vi "everything.vi"   [LabVIEW 2011]
uses:
  gfitsio.lvlib
  cfitsio-hdutypes.ctl
  gfitsio-error-codes.ctl
  gfitsio-refnum.ctl
  cfitsio-bitpix.ctl
types:
  T1 = typedef "gfitsio.lvlib/gfitsio-refnum.ctl" = refnum<k1>
  T2 = typedef "gfitsio.lvlib/cfitsio-hdutypes.ctl" = i32
  T3 = typedef "gfitsio.lvlib/gfitsio-error-codes.ctl" = i32
  T4 = typedef "gfitsio.lvlib/cfitsio-bitpix.ctl" = i32
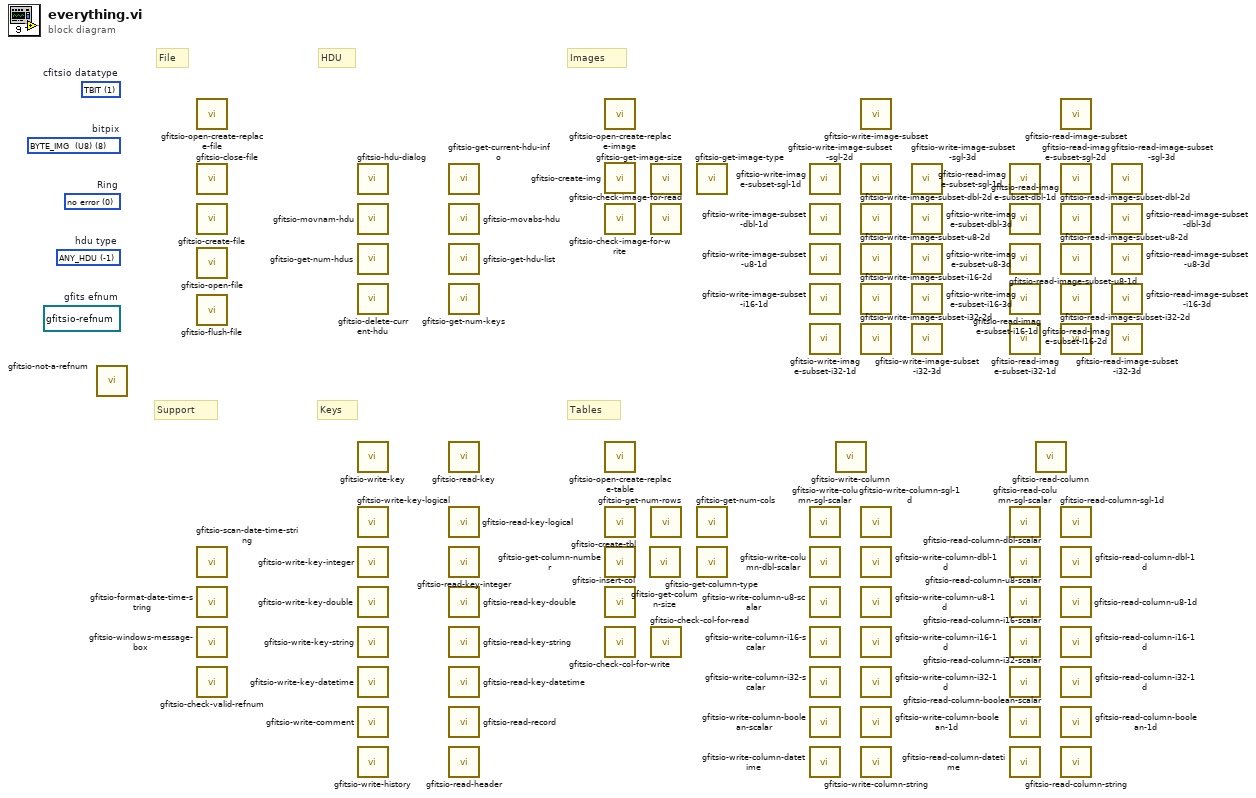
[diagram p0: block diagram]
diagram:
  (unwired) T1 refnum items=["GFITSIO"]  # gfits efnum
  (unwired) T2 -1 items=["ANY_HDU"=-1, "IMAGE_HDU"=0, "ASCII_TBL"=1, "BINARY_TBL"=2]  # hdu type
  (unwired) T3 0 items=["no error"=0, "dimensionality conflict"=5001, "fpixel out of image bounds"=5002, "lpixel out of image bounds"=5003, "increment size larger than image"=5004, "increment must be greater than zero"=5005, "fpixel must specify lower left corner"=5006, "named HDU not found"=5007, "specified row is past the end of the table"=5008, "wrong number of elements for column"=5009, "column is not scalar"=5010, "duplicate HDU name"=5011, "invalid table type"=5012]  # Ring
  (unwired) T4 8 items=["<invalid type>"=0, "BYTE_IMG  (U8)"=8, "SHORT_IMG  (I16)"=16, "USHORT_IMG  (U16)"=20, "LONG_IMG  (I32)"=32, "ULONG_IMG  (U32)"=40, "FLOAT_IMG  (SGL)"=-32, "DOUBLE_IMG  (DBL)"=-64]  # bitpix
  (unwired) T2 1 items=["TBIT"=1, "TBYTE  (U8)"=11, "TSBYTE  (I8)"=12, "TLOGICAL"=14, "TSTRING"=16, "TUSHORT  (U16)"=20, "TSHORT  (I16)"=21, "TUINT"=31, "TULONG  (U32)"=40, "TLONG  (I32)"=41, "TFLOAT  (SGL)"=42, "TLONGLONG  (I64)"=81, "TDOUBLE  (DBL)"=82, "TCOMPLEX  (CSG)"=83, "TDOUBLECOMPLEX  (CDB)"=163]  # cfitsio datatype
  # "Tables"
  # "Keys"
  # "Support"
  # "Images"
  # "HDU"
  # "File"
  n1 = call "gfitsio-not-a-refnum.vi"() -> ()  [unwired: 1 out]
  n2 = call "gfitsio-open-create-replace-file.vi"() -> ()  [unwired: 9 in, 3 out]
  n3 = call "gfitsio-close-file.vi"() -> ()  [unwired: 10 in, 2 out]
  n4 = call "gfitsio-create-file.vi"() -> ()  [unwired: 10 in, 2 out]
  n5 = call "gfitsio-open-file.vi"() -> ()  [unwired: 10 in, 2 out]
  n6 = call "gfitsio-flush-file.vi"() -> ()  [unwired: 10 in, 2 out]
  n7 = call "gfitsio-scan-date-time-string.vi"() -> ()  [unwired: 10 in, 2 out]
  n8 = call "gfitsio-format-date-time-string.vi"() -> ()  [unwired: 11 in, 1 out]
  n9 = call "gfitsio-windows-message-box.vi"() -> ()  [unwired: 11 in, 1 out]
  n10 = call "gfitsio-check-valid-refnum.vi"() -> ()  [unwired: 5 in, 1 out]
  n11 = call "gfitsio-hdu-dialog.vi"() -> ()  [unwired: 6 in, 6 out]
  n12 = call "gfitsio-movnam-hdu.vi"() -> ()  [unwired: 10 in, 2 out]
  n13 = call "gfitsio-get-num-hdus.vi"() -> ()  [unwired: 9 in, 3 out]
  n14 = call "gfitsio-delete-current-hdu.vi"() -> ()  [unwired: 10 in, 2 out]
  n15 = call-poly "gfitsio-write-key.vi"() -> ()  [unwired: 10 in, 2 out]
  n16 = call "gfitsio-write-key-logical.vi"() -> ()  [unwired: 10 in, 2 out]
  n17 = call "gfitsio-write-key-integer.vi"() -> ()  [unwired: 10 in, 2 out]
  n18 = call "gfitsio-write-key-double.vi"() -> ()  [unwired: 10 in, 2 out]
  n19 = call "gfitsio-write-key-string.vi"() -> ()  [unwired: 10 in, 2 out]
  n20 = call "gfitsio-write-key-datetime.vi"() -> ()  [unwired: 10 in, 2 out]
  n21 = call "gfitsio-write-comment.vi"() -> ()  [unwired: 10 in, 2 out]
  n22 = call "gfitsio-write-history.vi"() -> ()  [unwired: 10 in, 2 out]
  n23 = call "gfitsio-get-current-hdu-info.vi"() -> ()  [unwired: 7 in, 5 out]
  n24 = call "gfitsio-movabs-hdu.vi"() -> ()  [unwired: 9 in, 3 out]
  n25 = call "gfitsio-get-hdu-list.vi"() -> ()  [unwired: 8 in, 4 out]
  n26 = call "gfitsio-get-num-keys.vi"() -> ()  [unwired: 9 in, 3 out]
  n27 = call-poly "gfitsio-read-key.vi"() -> ()  [unwired: 7 in, 5 out]
  n28 = call "gfitsio-read-key-logical.vi"() -> ()  [unwired: 8 in, 4 out]
  n29 = call "gfitsio-read-key-integer.vi"() -> ()  [unwired: 7 in, 5 out]
  n30 = call "gfitsio-read-key-double.vi"() -> ()  [unwired: 7 in, 5 out]
  n31 = call "gfitsio-read-key-string.vi"() -> ()  [unwired: 8 in, 4 out]
  n32 = call "gfitsio-read-key-datetime.vi"() -> ()  [unwired: 8 in, 4 out]
  n33 = call "gfitsio-read-record.vi"() -> ()  [unwired: 9 in, 3 out]
  n34 = call "gfitsio-read-header.vi"() -> ()  [unwired: 9 in, 3 out]
  n35 = call "gfitsio-open-create-replace-image.vi"() -> ()  [unwired: 9 in, 3 out]
  n36 = call "gfitsio-create-img.vi"() -> ()  [unwired: 10 in, 2 out]
  n37 = call "gfitsio-check-image-for-write.vi"() -> ()  [unwired: 10 in, 2 out]
  n38 = call "gfitsio-open-create-replace-table.vi"() -> ()  [unwired: 9 in, 3 out]
  n39 = call "gfitsio-create-tbl.vi"() -> ()  [unwired: 10 in, 2 out]
  n40 = call "gfitsio-get-column-number.vi"() -> ()  [unwired: 9 in, 3 out]
  n41 = call "gfitsio-insert-col.vi"() -> ()  [unwired: 10 in, 2 out]
  n42 = call "gfitsio-check-col-for-write.vi"() -> ()  [unwired: 9 in, 3 out]
  n43 = call "gfitsio-get-column-size.vi"() -> ()  [unwired: 8 in, 4 out]
  n44 = call "gfitsio-get-image-size.vi"() -> ()  [unwired: 8 in, 4 out]
  n45 = call "gfitsio-check-image-for-read.vi"() -> ()  [unwired: 9 in, 3 out]
  n46 = call "gfitsio-get-num-rows.vi"() -> ()  [unwired: 9 in, 3 out]
  n47 = call "gfitsio-check-col-for-read.vi"() -> ()  [unwired: 9 in, 3 out]
  n48 = call "gfitsio-get-image-type.vi"() -> ()  [unwired: 9 in, 3 out]
  n49 = call "gfitsio-get-num-cols.vi"() -> ()  [unwired: 9 in, 3 out]
  n50 = call "gfitsio-get-column-type.vi"() -> ()  [unwired: 8 in, 4 out]
  n51 = call "gfitsio-write-image-subset-sgl-1d.vi"() -> ()  [unwired: 10 in, 2 out]
  n52 = call "gfitsio-write-image-subset-dbl-1d.vi"() -> ()  [unwired: 10 in, 2 out]
  n53 = call "gfitsio-write-image-subset-u8-1d.vi"() -> ()  [unwired: 10 in, 2 out]
  n54 = call "gfitsio-write-image-subset-i16-1d.vi"() -> ()  [unwired: 10 in, 2 out]
  n55 = call "gfitsio-write-image-subset-i32-1d.vi"() -> ()  [unwired: 10 in, 2 out]
  n56 = call "gfitsio-write-column-sgl-scalar.vi"() -> ()  [unwired: 10 in, 2 out]
  n57 = call "gfitsio-write-column-dbl-scalar.vi"() -> ()  [unwired: 10 in, 2 out]
  n58 = call "gfitsio-write-column-u8-scalar.vi"() -> ()  [unwired: 10 in, 2 out]
  n59 = call "gfitsio-write-column-i16-scalar.vi"() -> ()  [unwired: 10 in, 2 out]
  n60 = call "gfitsio-write-column-i32-scalar.vi"() -> ()  [unwired: 10 in, 2 out]
  n61 = call "gfitsio-write-column-boolean-scalar.vi"() -> ()  [unwired: 10 in, 2 out]
  n62 = call "gfitsio-write-column-datetime.vi"() -> ()  [unwired: 10 in, 2 out]
  n63 = call-poly "gfitsio-write-column.vi"() -> ()  [unwired: 10 in, 2 out]
  n64 = call-poly "gfitsio-write-image-subset.vi"() -> ()  [unwired: 10 in, 2 out]
  n65 = call "gfitsio-write-image-subset-sgl-2d.vi"() -> ()  [unwired: 10 in, 2 out]
  n66 = call "gfitsio-write-image-subset-dbl-2d.vi"() -> ()  [unwired: 10 in, 2 out]
  n67 = call "gfitsio-write-image-subset-u8-2d.vi"() -> ()  [unwired: 10 in, 2 out]
  n68 = call "gfitsio-write-image-subset-i16-2d.vi"() -> ()  [unwired: 10 in, 2 out]
  n69 = call "gfitsio-write-image-subset-i32-2d.vi"() -> ()  [unwired: 10 in, 2 out]
  n70 = call "gfitsio-write-column-sgl-1d.vi"() -> ()  [unwired: 10 in, 2 out]
  n71 = call "gfitsio-write-column-dbl-1d.vi"() -> ()  [unwired: 10 in, 2 out]
  n72 = call "gfitsio-write-column-u8-1d.vi"() -> ()  [unwired: 10 in, 2 out]
  n73 = call "gfitsio-write-column-i16-1d.vi"() -> ()  [unwired: 10 in, 2 out]
  n74 = call "gfitsio-write-column-i32-1d.vi"() -> ()  [unwired: 10 in, 2 out]
  n75 = call "gfitsio-write-column-boolean-1d.vi"() -> ()  [unwired: 10 in, 2 out]
  n76 = call "gfitsio-write-column-string.vi"() -> ()  [unwired: 10 in, 2 out]
  n77 = call "gfitsio-write-image-subset-sgl-3d.vi"() -> ()  [unwired: 10 in, 2 out]
  n78 = call "gfitsio-write-image-subset-dbl-3d.vi"() -> ()  [unwired: 10 in, 2 out]
  n79 = call "gfitsio-write-image-subset-u8-3d.vi"() -> ()  [unwired: 10 in, 2 out]
  n80 = call "gfitsio-write-image-subset-i16-3d.vi"() -> ()  [unwired: 10 in, 2 out]
  n81 = call "gfitsio-write-image-subset-i32-3d.vi"() -> ()  [unwired: 10 in, 2 out]
  n82 = call "gfitsio-read-image-subset-sgl-1d.vi"() -> ()  [unwired: 8 in, 4 out]
  n83 = call "gfitsio-read-image-subset-dbl-1d.vi"() -> ()  [unwired: 8 in, 4 out]
  n84 = call "gfitsio-read-image-subset-u8-1d.vi"() -> ()  [unwired: 8 in, 4 out]
  n85 = call "gfitsio-read-image-subset-i16-1d.vi"() -> ()  [unwired: 8 in, 4 out]
  n86 = call "gfitsio-read-image-subset-i32-1d.vi"() -> ()  [unwired: 8 in, 4 out]
  n87 = call "gfitsio-read-column-sgl-scalar.vi"() -> ()  [unwired: 9 in, 3 out]
  n88 = call "gfitsio-read-column-dbl-scalar.vi"() -> ()  [unwired: 9 in, 3 out]
  n89 = call "gfitsio-read-column-u8-scalar.vi"() -> ()  [unwired: 9 in, 3 out]
  n90 = call "gfitsio-read-column-i16-scalar.vi"() -> ()  [unwired: 9 in, 3 out]
  n91 = call "gfitsio-read-column-i32-scalar.vi"() -> ()  [unwired: 9 in, 3 out]
  n92 = call "gfitsio-read-column-boolean-scalar.vi"() -> ()  [unwired: 9 in, 3 out]
  n93 = call "gfitsio-read-column-datetime.vi"() -> ()  [unwired: 9 in, 3 out]
  n94 = call-poly "gfitsio-read-column.vi"() -> ()  [unwired: 9 in, 3 out]
  n95 = call-poly "gfitsio-read-image-subset.vi"() -> ()  [unwired: 8 in, 4 out]
  n96 = call "gfitsio-read-image-subset-sgl-2d.vi"() -> ()  [unwired: 8 in, 4 out]
  n97 = call "gfitsio-read-image-subset-dbl-2d.vi"() -> ()  [unwired: 8 in, 4 out]
  n98 = call "gfitsio-read-image-subset-u8-2d.vi"() -> ()  [unwired: 8 in, 4 out]
  n99 = call "gfitsio-read-image-subset-I16-2d.vi"() -> ()  [unwired: 8 in, 4 out]
  n100 = call "gfitsio-read-image-subset-i32-2d.vi"() -> ()  [unwired: 8 in, 4 out]
  n101 = call "gfitsio-read-column-sgl-1d.vi"() -> ()  [unwired: 9 in, 3 out]
  n102 = call "gfitsio-read-column-dbl-1d.vi"() -> ()  [unwired: 9 in, 3 out]
  n103 = call "gfitsio-read-column-u8-1d.vi"() -> ()  [unwired: 9 in, 3 out]
  n104 = call "gfitsio-read-column-i16-1d.vi"() -> ()  [unwired: 9 in, 3 out]
  n105 = call "gfitsio-read-column-i32-1d.vi"() -> ()  [unwired: 9 in, 3 out]
  n106 = call "gfitsio-read-column-boolean-1d.vi"() -> ()  [unwired: 9 in, 3 out]
  n107 = call "gfitsio-read-column-string.vi"() -> ()  [unwired: 9 in, 3 out]
  n108 = call "gfitsio-read-image-subset-sgl-3d.vi"() -> ()  [unwired: 8 in, 4 out]
  n109 = call "gfitsio-read-image-subset-dbl-3d.vi"() -> ()  [unwired: 8 in, 4 out]
  n110 = call "gfitsio-read-image-subset-u8-3d.vi"() -> ()  [unwired: 8 in, 4 out]
  n111 = call "gfitsio-read-image-subset-i16-3d.vi"() -> ()  [unwired: 8 in, 4 out]
  n112 = call "gfitsio-read-image-subset-i32-3d.vi"() -> ()  [unwired: 8 in, 4 out]
